vi "Memory.Pointer.I32.New.vi"(8 "error in (no error)":errorcluster, 10 "count (1)":u64=1, 11 "I32 Pointer in":refnum<class "Memory.Pointer.I32.lvclass">) -> (0 "error out":errorcluster, 3 "I32 Pointer out":refnum<class "Memory.Pointer.I32.lvclass">)   [LabVIEW 2016, in "Memory.lvlib" / "Memory.Pointer.I32.lvclass"]
uses:
  Memory.Pointer.I32.lvclass
  C:/Git/Sourcetree/DSF/Source/Submodules/Memory/Source/Classes/Internal/Memory.Pointer.Internal.lvclass
  Internal/Memory.Pointer.Internal.New.4B.vi
  Internal/Memory.Pointer.Internal.Allocate.vi
  Internal/Memory.Pointer.Internal.lvclass
  C:/Git/Sourcetree/DSF/Source/Submodules/Memory/Source/Classes/Pointer/Memory.Pointer.lvclass
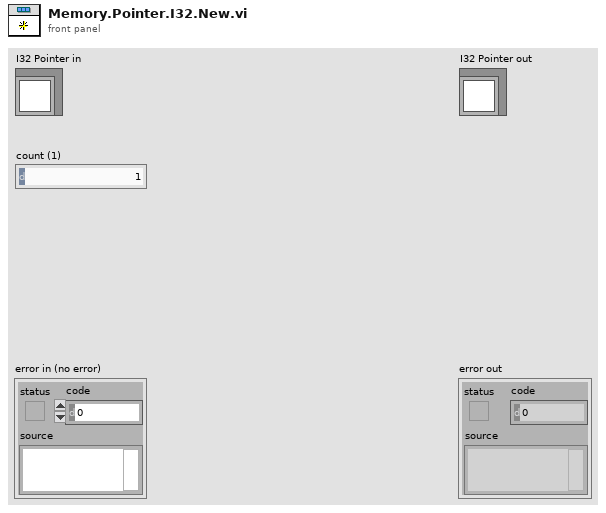
[diagram p1: front panel]
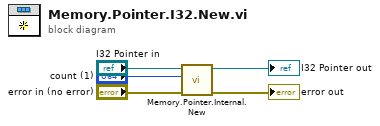
[diagram p0: block diagram]
diagram:
  n1 = call-poly "Memory.Pointer.Internal.New.vi"("error in (no error)"="error in (no error)", "count (1)"="count (1)", "pointer type"="I32 Pointer in") -> ("error out"=→"error out":errorcluster, "pointer out"=→"I32 Pointer out":refnum<class "Memory.Pointer.I32.lvclass">)  [unwired: 7 in]
